vi "ExecutionFrequency.vi"(11 "Moving Average Length":i32) -> (1 "Timestamp (s)":dbl format="%.8f", 2 "Frequency (Hz)":dbl, 3 "Period (s)":dbl)   [LabVIEW 2014]
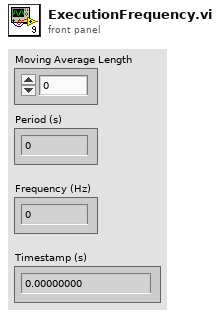
[diagram p1: front panel]
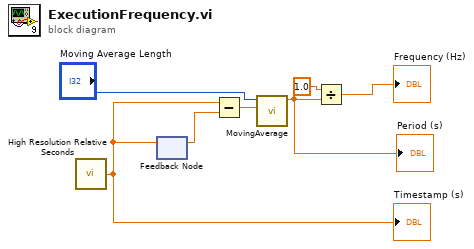
[diagram p0: block diagram]
diagram:
  n1 = call <vilib>:"High Resolution Relative Seconds.vi"() -> ("relative seconds"=w7:dbl)
  "Timestamp (s)" <- w7
  n2 = feedback #1() -> (w5:dbl)  [unwired: 1 in]
  n3 = feedback-in #1(w7) -> ()
  n4 = Subtract(x=w7, y=w5) -> (x-y=w3:dbl)
  n5 = call "MovingAverage.vi"("Datapoint"=w3, "Moving Average Length"="Moving Average Length") -> ("Moving Average"=w1:dbl)  [unwired: 9 in]
  "Period (s)" <- w1
  n6 = Divide(x=1.0, y=w1) -> (x/y=→"Frequency (Hz)":dbl)
